vi "Control Servo.vi"(8 "error in (no error)":errorcluster, 9 "setpoint":dbl, 10 "process variable":dbl, 11 "Open-loop Controller in":refnum<class "Open-loop Controller.lvclass">) -> (0 "error out":errorcluster, 2 "servo pw (us)":dbl, 3 "Open-loop Controller out":refnum<class "Open-loop Controller.lvclass">)   [LabVIEW 2020, in "Open-loop Controller.lvclass"]
uses:
  Open-loop Controller.lvclass
  Open-loop Controller.lvclass/Open-loop Controller.ctl
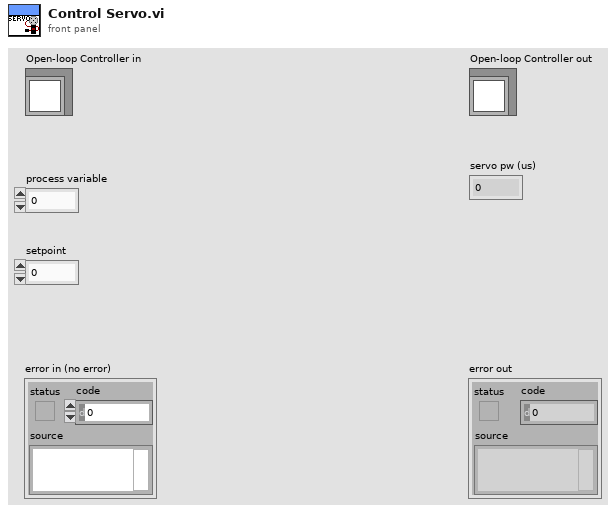
[diagram p1: front panel]
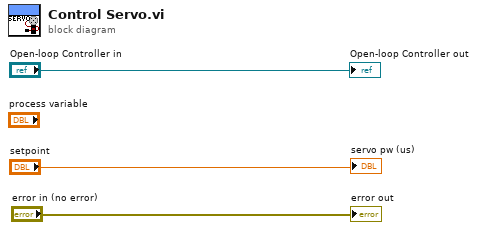
[diagram p0: block diagram]
diagram:
  "error out" <- "error in (no error)"
  "Open-loop Controller out" <- "Open-loop Controller in"
  "servo pw (us)" <- "setpoint"
